vi "MRU Example.vi"() -> ()   [LabVIEW 2014]
uses:
  MRU.lvclass
panel:
  out "INI File Contents":string
  in  "Say It":bool
  in  "Message":string(combo)
  # "This VI demonstrates the use of the MRU library.\n\n    The MRU library is designed to quickly and easily automate synchronization of a 'Most Recently\nUsed' list between a System Combo Box and an INI file.\n\n    How to use this example:\n1. Ensure it exists in a folder that LabVIEW has Read/Write Access\n2. Run the VI\n3. Enter some text in the Message combo box and hit the Say It button\n4. Hit OK on the dialog that shows\n5. Repeat steps 3-4 while observing the INI File Contents indicator\n6. Close the VI using the X (not the Stop/Abort button)"
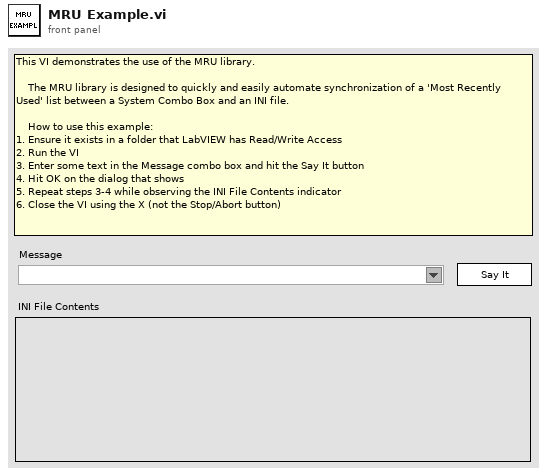
[diagram p1: front panel]
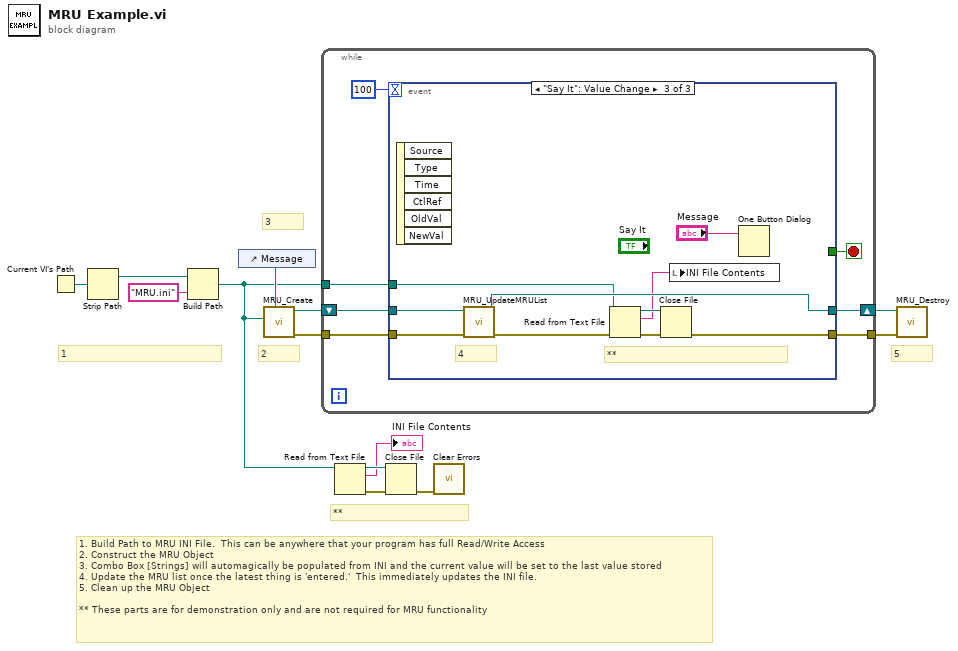
[diagram p0: block diagram]
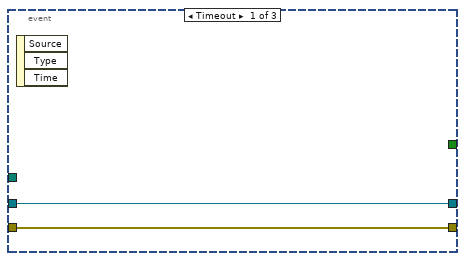
[diagram p2: hidden frame]
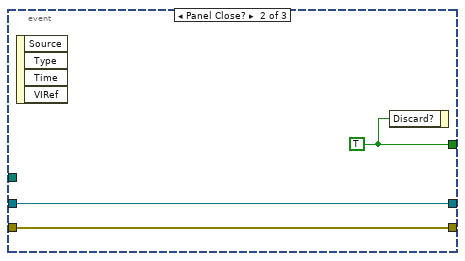
[diagram p3: hidden frame]
diagram:
  # "**"
  # "5"
  # "3"
  # "2"
  # "1"
  # "1. Build Path to MRU INI File.  This can be anywhere that your program has full Read/Write Access\n2. Construct the MRU Object\n3. Combo Box [Strings] will automagically be populated from INI and the current value will be set to the last value stored\n4. Update the MRU list once the latest thing is 'entered.'  This immediately updates the INI file.\n5. Clean up the MRU Object\n\n** These parts are for demonstration only and are not required for MRU functionality"
  n1 = Current VI's Path() -> (path=w13:path)
  n2 = Strip Path(path=w13) -> (stripped path=w12:path)  [unwired: 1 out]
  n3 = Build Path(base path=w12, name or relative path="MRU.ini") -> (appended path=w3:path)
  n4 = control-ref of="Message"() -> (w10:refnum<vi>)
  n5 = call "MRU_Create.vi"("CmbBox Refnum"=w10, "MRU INI file (c:\\mru.ini)"=w3) -> ("error out"=w9:errorcluster, "reference out"=w8:refnum<class "MRU.lvclass">)  [unwired: 8 in]
  n6 = while {
    tunnel: w9 -> [w19]
    shift-right: [w18] -> w7
    shift-left: w8 -> [w20]
    tunnel: [w17] -> w6
    tunnel: w3 -> [w14]
    stop <- w16 stop-if-true
    n7 = event shown="[2] \"Say It\": Value Change" {
      selector: _ -> [_ _ _]
      dyn-events: _ -> [_ _ _]
      timeout: 100 -> [_ _ _]
      tunnel: w20 -> [w22 w25 w34]
      tunnel: w19 -> [w21 w24 w35]
      tunnel: [w22 w25 w31] -> w18
      tunnel: [w21 w24 w28] -> w17
      tunnel: [_ w23 _] -> w16
      tunnel: w14 -> [_ _ w29]
      event Timeout {
        n8 = event-data() -> ()  [unwired: 1 in, 3 out]
      }
      event Panel Close? {
        w23 = TRUE ("Discard?")
        n9 = event-data() -> ()  [unwired: 1 in, 4 out]
        n10 = event-data("Discard?"=w23) -> ()  [unwired: 1 in, 1 out]
      }
      event "Say It": Value Change {
        # "**"
        # "4"
        n11 = event-data() -> ()  [unwired: 1 in, 6 out]
        n12 = call-dynamic "MRU_UpdateMRUList.vi"("error in (no error)"=w35, "reference in"=w34) -> ("error out"=w33:errorcluster, "reference out"=w31:refnum<class "MRU.lvclass">)  [unwired: 8 in]
        n13 = Read from Text File(file (use dialog)=w29, error in=w33) -> (refnum out=w27:refnum<file>, text=w26:string, error out=w30:errorcluster)  [unwired: 2 in, 1 out]
        n14 = Close File(refnum=w27, error in=w30) -> (error out=w28:errorcluster)  [unwired: 1 out]
        n15 = local write "INI File Contents"(w26) -> ()
        n16 = One Button Dialog(message="Message") -> ()  [unwired: 1 in, 1 out]
      }
    }
  }
  n17 = Read from Text File(file (use dialog)=w3) -> (refnum out=w5:refnum<file>, text=→"INI File Contents":string, error out=w4:errorcluster)  [unwired: 3 in, 1 out]
  n18 = Close File(refnum=w5, error in=w4) -> (error out=w1:errorcluster)  [unwired: 1 out]
  n19 = call <vilib>:"Clear Errors.vi"("error in (no error)"=w1) -> ()  [unwired: 5 in, 2 out]
  n20 = call-dynamic "MRU_Destroy.vi"("error in (no error)"=w6, "reference in"=w7) -> ()  [unwired: 8 in, 2 out]
